vi "GetPaths.vi"() -> (2 "Paths":T1)   [LabVIEW 2020, in "Pin_Instrument_Factory.lvclass"]
uses:
  Pin_Instrument_Factory.lvclass
  Typedefs/Paths.ctl
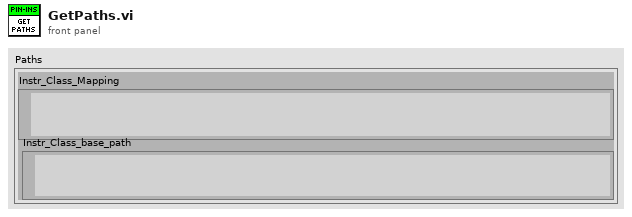
[diagram p1: front panel]
types:
  T1 = typedef "Pin_Instrument_Factory.lvclass/Paths.ctl" = cluster{"Instr_Class_Mapping":path, "Instr_Class_base_path":path}
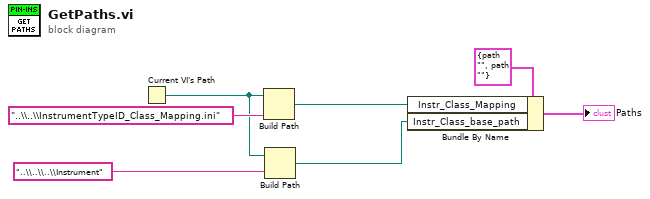
[diagram p0: block diagram]
diagram:
  n1 = Current VI's Path() -> (path=w3:path)
  n2 = Build Path(base path=w3, name or relative path="..\\..\\InstrumentTypeID_Class_Mapping.ini") -> (appended path=w5:path)
  n3 = Build Path(base path=w3, name or relative path="..\\..\\..\\Instrument") -> (appended path=w1:path)
  n4 = Bundle By Name(cluster=T1 {"Instr_Class_Mapping"=path "", "Instr_Class_base_path"=path ""}, "Instr_Class_Mapping"=w5, "Instr_Class_base_path"=w1) -> (→"Paths":T1)
